vi "CalcVoltLabel.vi"(1 "InputVolt":dbl format="%#_13g") -> (0 "VoltString":string)   [LabVIEW 2015, in "CS++ScopeGui.lvlib" / "CS++ScopeGui.lvclass"]
doc: "Small conversion needed inside the ActorCore"
uses:
  CS++ScopeGui.lvclass
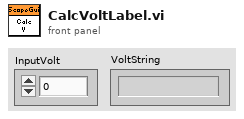
[diagram p1: front panel]
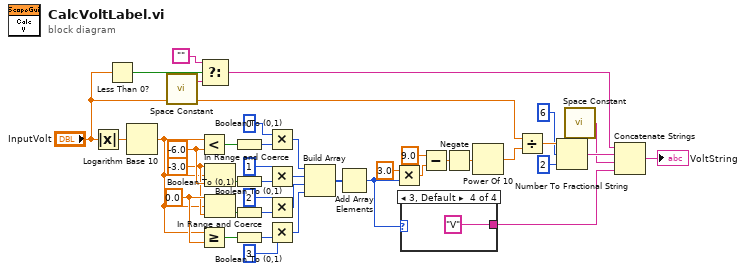
[diagram p0: block diagram]
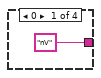
[diagram p2: hidden frame]
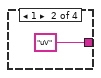
[diagram p3: hidden frame]
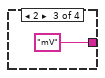
[diagram p4: hidden frame]
diagram:
  w40 = 0.0 ("upper limit")
  w24 = -3.0 ("y")
  w41 = -6.0 ("y")
  n1 = Absolute Value(x="InputVolt") -> (abs(x)=w7:dbl)
  n2 = Less Than 0?(x="InputVolt") -> (x < 0?=w4:bool)
  n3 = Logarithm Base 10(1:w7) -> (0:w21:dbl)
  n4 = call <vilib>:"Space Constant.vi"() -> ("String"=w1:string)
  n5 = Less?(x=w21, y=w41) -> (x < y?=w39:bool)
  n6 = Greater Or Equal?(x=w21, y=w40) -> (x >= y?=w36:bool)
  n7 = Select(t="", s=w4, f=w1) -> (s? t:f=w2:string)
  n8 = In Range and Coerce(upper limit=w24, x=w21, lower limit=w41) -> (In Range?=w38:bool)  [unwired: 1 out]
  n9 = In Range and Coerce(upper limit=w40, x=w21, lower limit=w24) -> (In Range?=w37:bool)  [unwired: 1 out]
  n10 = Boolean To (0,1)(Boolean=w39) -> (0, 1=w32:i16)
  n11 = Boolean To (0,1)(Boolean=w38) -> (0, 1=w33:i16)
  n12 = Boolean To (0,1)(Boolean=w37) -> (0, 1=w34:i16)
  n13 = Boolean To (0,1)(Boolean=w36) -> (0, 1=w35:i16)
  n14 = Multiply(x=i16 0, y=w32) -> (x*y=w28:i16)
  n15 = Multiply(x=i16 1, y=w33) -> (x*y=w27:i16)
  n16 = Multiply(x=i16 2, y=w34) -> (x*y=w26:i16)
  n17 = Multiply(x=i16 3, y=w35) -> (x*y=w25:i16)
  n18 = Build Array(w28, w27, w26, w25) -> (w22:i16[])
  n19 = Add Array Elements(numeric array=w22) -> (sum=w15:i16)
  n20 = Multiply(x=3.0, y=w15) -> (x*y=w18:dbl)
  n21 = case shown="3, Default" w15 {
    tunnel: ["nV" ("string") "uV" ("string") "mV" ("string") "V" ("string")] -> w9
    frame 0 {
    }
    frame 1 {
    }
    frame 2 {
    }
    frame 3, Default {
    }
  }
  n22 = Subtract(x=9.0, y=w18) -> (x-y=w17:dbl)
  n23 = Negate(x=w17) -> (-x=w16:dbl)
  n24 = Power Of 10(x=w16) -> (10^x=w14:dbl)
  n25 = Divide(x="InputVolt", y=w14) -> (x/y=w12:dbl)
  n26 = Number To Fractional String(number=w12, width (-)=i16 6, precision (6)=i16 2) -> (F-format string=w11:string)  [unwired: 1 in]
  n27 = call <vilib>:"Space Constant.vi"() -> ("String"=w8:string)
  n28 = Concatenate Strings(w2, w11, w8, w9) -> (→"VoltString":string)
